vi "get network devices.vi"(6 "local subnet only (T)":bool caption="Local Subnet Only (F)", 8 "error in":errorcluster, 9 "device class string":string[](array[string]), 10 "device class":T1, 11 "syscfg device in":refnum<class "SysCfg Device.lvclass">) -> (0 "error out":errorcluster, 2 "devices":T2[](array[typedef]) {"product ID" format="%.0x"}, 3 "syscfg device out":refnum<class "SysCfg Device.lvclass">)   [LabVIEW 2014, in "SMI.lvlib" / "SysCfg Device.lvclass"]
uses:
  SysCfg Device.lvclass
  Device/network device information.ctl
  Device/device class selection.ctl
  Device/Device.lvclass
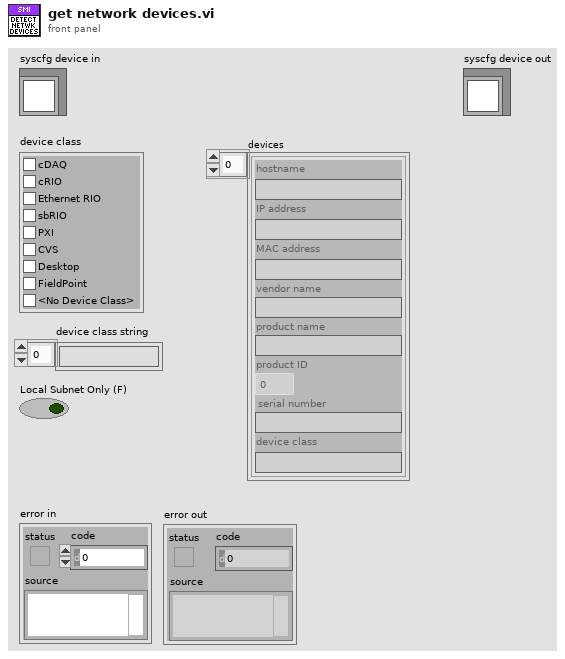
[diagram p1: front panel]
types:
  T1 = typedef "SMI.lvlib/Device.lvclass/device class selection.ctl" = cluster{"cDAQ":bool, "cRIO":bool, "Ethernet RIO":bool, "sbRIO":bool, "PXI":bool, "CVS":bool, "Desktop":bool, "FieldPoint":bool, "<No Device Class>":bool}
  T2 = typedef "SMI.lvlib/Device.lvclass/network device information.ctl" = cluster{"hostname":string, "IP address":string, "MAC address":string, "vendor name":string, "product name":string, "product ID":u16, "serial number":string, "device class":string}
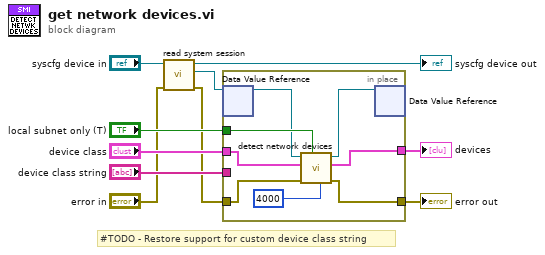
[diagram p0: block diagram]
diagram:
  # "#TODO - Restore support for custom device class string"
  n1 = call "read system session.vi"("error in"="error in", "syscfg device in"="syscfg device in") -> ("error out"=w2:errorcluster, "system session"=w4:refnum<data-value>, "syscfg device out"=→"syscfg device out":refnum<class "SysCfg Device.lvclass">)  [unwired: 7 in]
  n2 = in-place {
    in-place-border: "local subnet only (T)" -> [w18]
    in-place-border: w2 -> [w16]
    in-place-border: [w15] -> w10
    in-place-border: "device class string" -> [_]
    in-place-border: "device class" -> [w14]
    in-place-border: [w13] -> w9
    n3 = in-place-dvr #1(w4) -> (w12:refnum<k21>)  [unwired: 1 out]
    n4 = call "detect network devices.vi"("remote timeout (300,000 ms)"=u32 4000 ("Timeout (4000 ms)"), "local subnet only (F)"=w18, "error in"=w16, "device class"=w14, "system session (localhost)"=w12) -> ("error out"=w15:errorcluster, "devices"=w13:T2[], "system session out"=w11:refnum<k21>)  [unwired: 4 in]
    n5 = in-place-dvr #1(w11) -> ()  [unwired: 2 out]
  }
  "error out" <- w10
  "devices" <- w9
